vi "OP80FV_Check.vi"(6 "View":bool=TRUE, 8 "error in (no error)":errorcluster, 10 "RFID":string="0029032640C1845Ag000001", 11 "Ref in":T2={"MS SQL Connection"=refnum, "UDL File"=path "", "Time"="", "DCODE"="", "WIP+1"=0, "MC No?"=0, "POKAYOKE?"=FALSE, "Expected Result"="", "Result [Status]"="", "Clock"=0.0, "RFID"="", "WIP Queue"=refnum, "TS Parameter"={"ProfitCenterCode"="", "LineCode"="", "WorkOrderNumber"="", "Model"="", "Model_with_Prefix"="", "VendorCode"="", "SetParameterDateCode"="", "PokaYoke"=0, "Target"=1, "Live_DateCode"="", "CustomerPartNumber"="", "Hand"="", "sBarcode"=FALSE, "FCA"=0, "Ent_Stamp"=timestamp(0 s since 1904-01-01), "STS_CD"=0.0}, "Data_Queue"=[], "RFID Serial No."=""} {"TS Parameter"."FCA" format="%01d"; "TS Parameter"."Target" min=1 max=100000; "TS Parameter"."PokaYoke" min=0 max=1}) -> (0 "error out":errorcluster, 1 "Fail?":bool=TRUE, 2 "Pass?":bool=TRUE, 3 "Ref Out":T2={"MS SQL Connection"=refnum, "UDL File"=path "", "Time"="", "DCODE"="", "WIP+1"=0, "MC No?"=0, "POKAYOKE?"=FALSE, "Expected Result"="", "Result [Status]"="", "Clock"=0.0, "RFID"="", "WIP Queue"=refnum, "TS Parameter"={"ProfitCenterCode"="", "LineCode"="", "WorkOrderNumber"="", "Model"="", "Model_with_Prefix"="", "VendorCode"="", "SetParameterDateCode"="", "PokaYoke"=0, "Target"=1, "Live_DateCode"="", "CustomerPartNumber"="", "Hand"="", "sBarcode"=FALSE, "FCA"=0, "Ent_Stamp"=timestamp(0 s since 1904-01-01), "STS_CD"=0.0}, "Data_Queue"=[], "RFID Serial No."=""} {"TS Parameter"."FCA" format="%01d"; "TS Parameter"."Target" min=1 max=100000; "TS Parameter"."PokaYoke" min=0 max=1}, 4 "Discard?":bool=TRUE, 5 "Reason Out":string, 7 "appended array":string[](array[string]))   [LabVIEW 2020]
uses:
  Controls/TD SQL.ctl
  <vilib>/addons/database/Connection.llb/Conn ObjectReference.ctl
  Controls/WIP_State.ctl
  Controls/TS_Parameter.ctl
  Controls/FV_Status.ctl
  <vilib>/Utility/miscctls.llb/LVPointTypeDef.ctl
  Controls/1775E_Authen_Level.ctl
  Controls/Station_Task.ctl
  MS SQL/MS_Global.vi
  <userlib>/_OpenG.lib/comparison/comparison.llb/Boolean Changed__ogtk.vi
  <userlib>/_OpenG.lib/comparison/comparison.llb/String Changed__ogtk.vi
  <vilib>/addons/database/Connection.llb/Conn Execute.vi
  <vilib>/addons/database/Recordset.llb/Rec Destroy - Connection.vi
  <vilib>/ethernetip/ethernetip.llb/EthernetIP Tag Write DINT.vi
  <vilib>/Utility/miscctls.llb/LVRowAndColumnTypeDef.ctl
  <vilib>/Utility/miscctls.llb/LVRowAndColumnUnsignedTypeDef.ctl
  <vilib>/ethernetip/ethernetip.lvlib
  <vilib>/addons/database/NI_Database_API.lvlib
panel:
  out "resulting string":string
  out "Barcode":string
  out "Text Command for Printer":string
  out "Last Printed BC Mirror":string
  out "Last Printed Barcode":string
  out "Numeric":i32
  in  "Hide":bool
  in  "Reprint":bool
  in  "Scan":bool
  out "OP80 RFID":string
  in  "Fail":bool
  out "Over all Status":T1 caption="Data Validation"
  in  "RH Barcode":string="0029032640C1845Ag000001"
  in  "LH Barcode":string="0029032640C1845Ag000001"
  out "pPASS":bool
  out "pFAIL":bool
  in  "Pass":bool caption="Final Viewing"
  in  "Report":i32(listbox)
  in  "Time to Close":dbl format="%.1f"
  in  "Reason":string
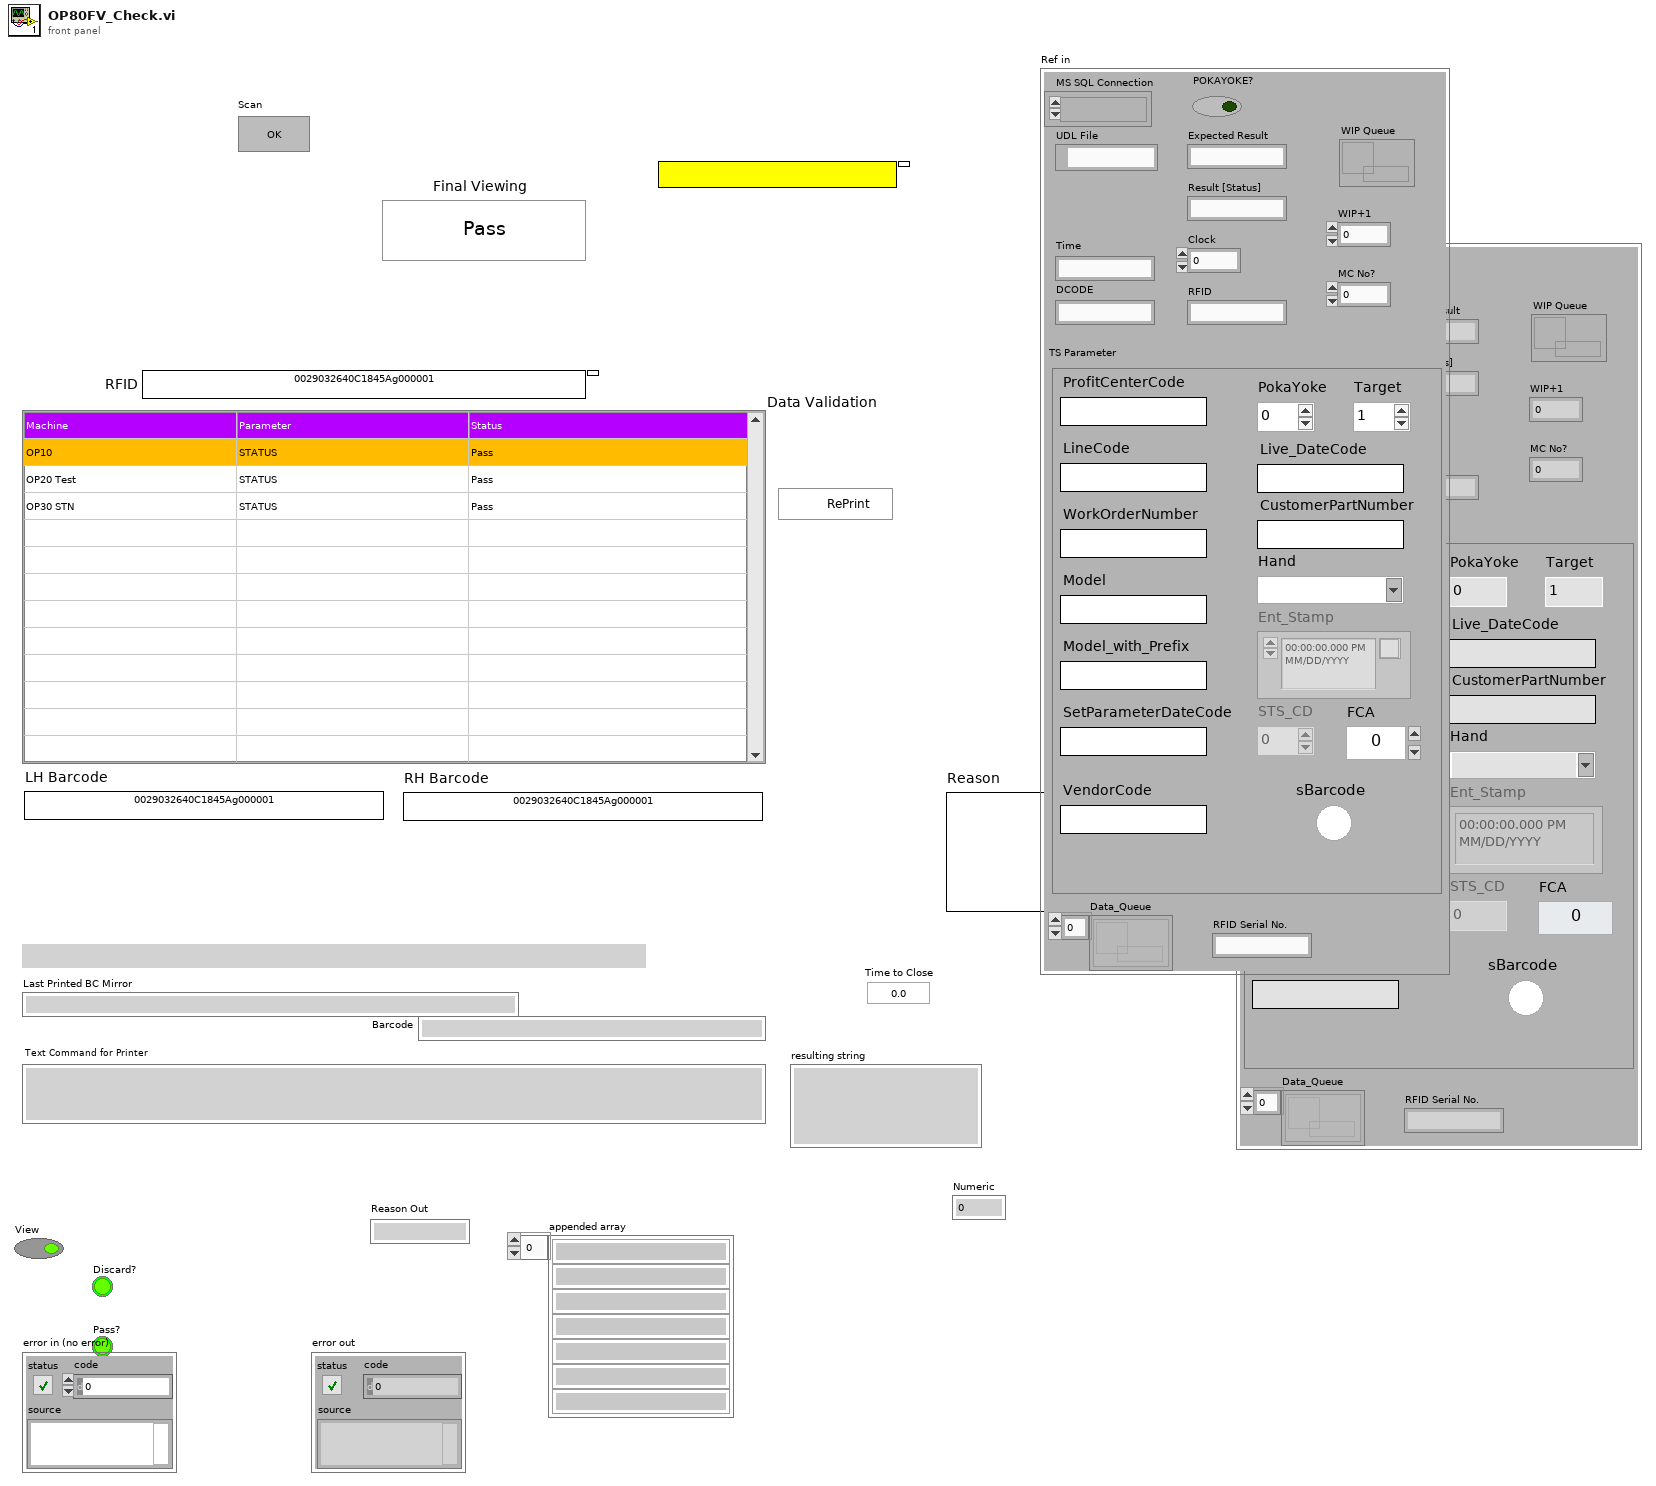
[diagram p1: front panel]
types:
  T1 = typedef "FV_Status.ctl" = u16
  T2 = typedef "TD SQL.ctl" = cluster{"MS SQL Connection":T3, "UDL File":path, "Time":string, "DCODE":string, "WIP+1":i64, "MC No?":i32, "POKAYOKE?":bool, "Expected Result":string, "Result [Status]":string, "Clock":dbl, "RFID":string, "WIP Queue":refnum<queue>, "TS Parameter":T4, "Data_Queue":refnum<queue>[], "RFID Serial No.":string}
  T3 = typedef "NI_Database_API.lvlib/Conn ObjectReference.ctl" = refnum<k1>
  T4 = typedef "TS_Parameter.ctl" = cluster{"ProfitCenterCode":string, "LineCode":string, "WorkOrderNumber":string, "Model":string, "Model_with_Prefix":string, "VendorCode":string, "SetParameterDateCode":string, "PokaYoke":i32, "Target":i32, "Live_DateCode":string, "CustomerPartNumber":string, "Hand":string, "sBarcode":bool, "FCA":i32, "Ent_Stamp":timestamp, "STS_CD":dbl}
  T5 = typedef "LVPointTypeDef.ctl" = cluster{"Horizontal":i16, "Vertical":i16}
  T6 = typedef "1775E_Authen_Level.ctl" = enum16{"Level 1", "Level 2", "Level 3", "Level 4", "Super Level"}
  T7 = typedef "LVRowAndColumnUnsignedTypeDef.ctl" = cluster{"Row":u32, "Column":u32}
  T8 = typedef "LVRowAndColumnTypeDef.ctl" = cluster{"Row":i32, "Column":i32}
  T9 = enum8{"Enabled", "Disabled", "Disabled and Grayed Out"}
  T10 = cluster{"CUSTOMER PART NUMBER":string, "Version Number":string, "VENDOR CODE":string, "BI PART NUMBER":string, "SCAN TYPE":enum16{"AUTO", "MANUAL"}, "BARCODE TYPE":enum16{"X451", "MSIL-YNC10 Trial1"}, "CELL NUMBER":string}
  T11 = typedef "Station_Task.ctl" = enum16{"Init", "Polling", "Check Bypass", "Check_Result", "get Barcode", "Pass", "Fail", "Check Data", "Log Data", "Idle_Alert", "DMS_Check", "FV_Check", "FV_View", "WRITE_RFID", "Exit"}
  T12 = typedef "user_log.ctl" = cluster{"eRID":u16, "eRName":string, "eRClock":string, "eRDate":timestamp, "eRLevel":string, "eRAdmin":string, "eRPassword":string}
  T13 = typedef "NI_Database_API.lvlib/Rec ObjectReference.ctl" = refnum<k1>
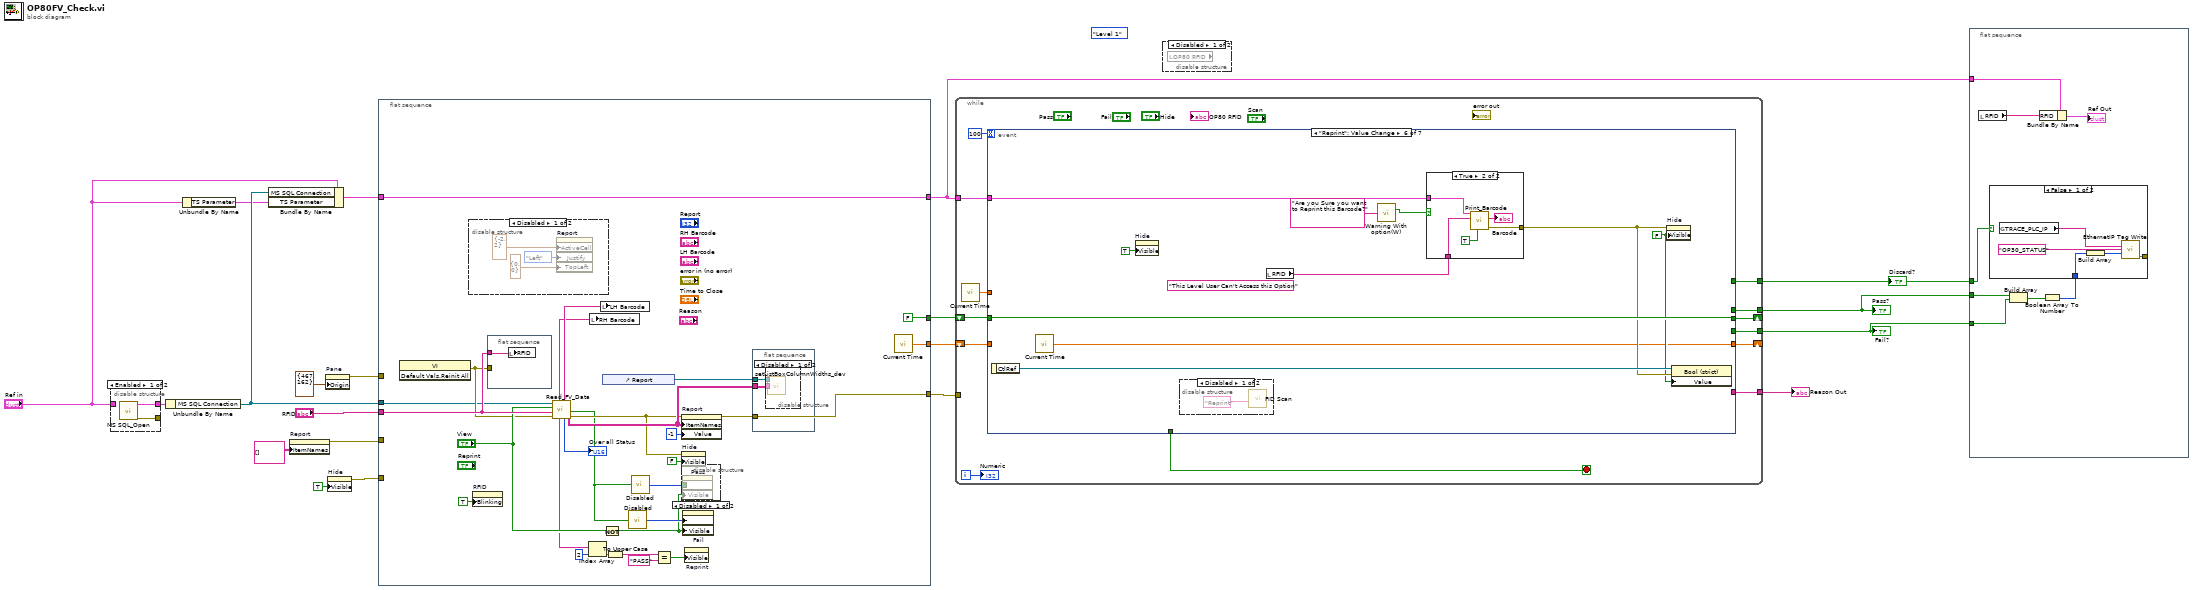
[diagram p0: block diagram]
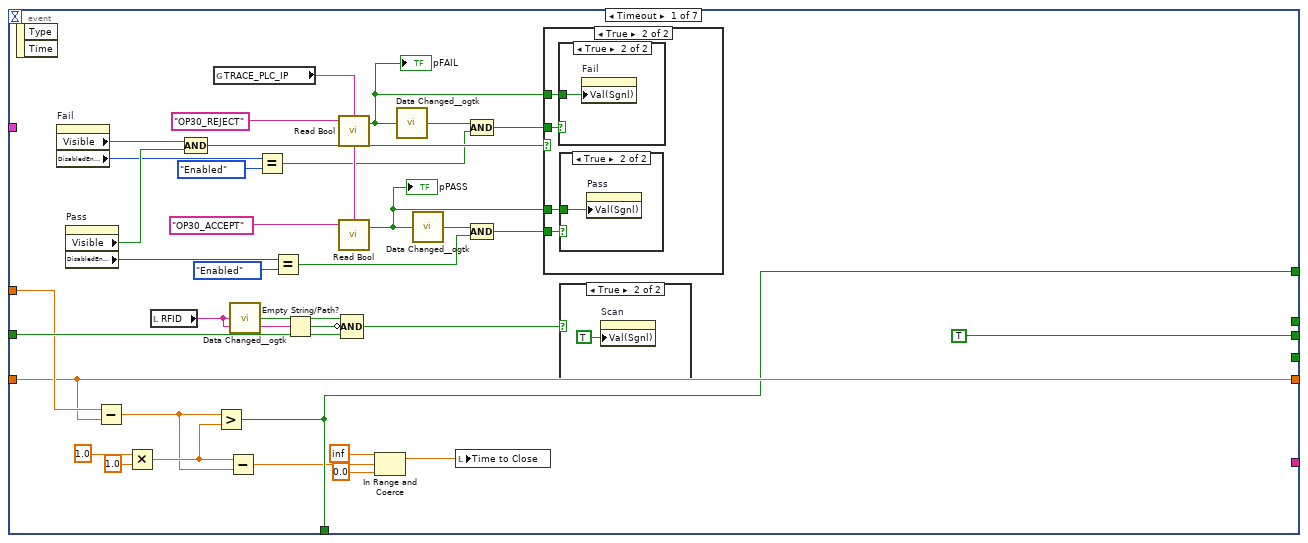
[diagram p8: hidden frame]
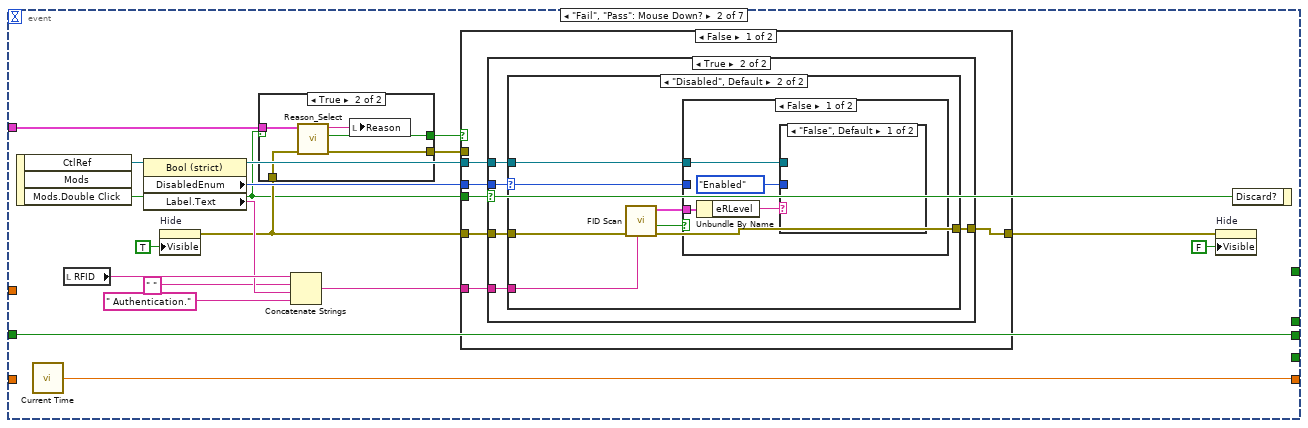
[diagram p13: hidden frame]
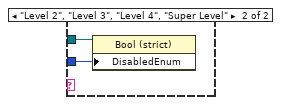
[diagram p17: hidden frame]
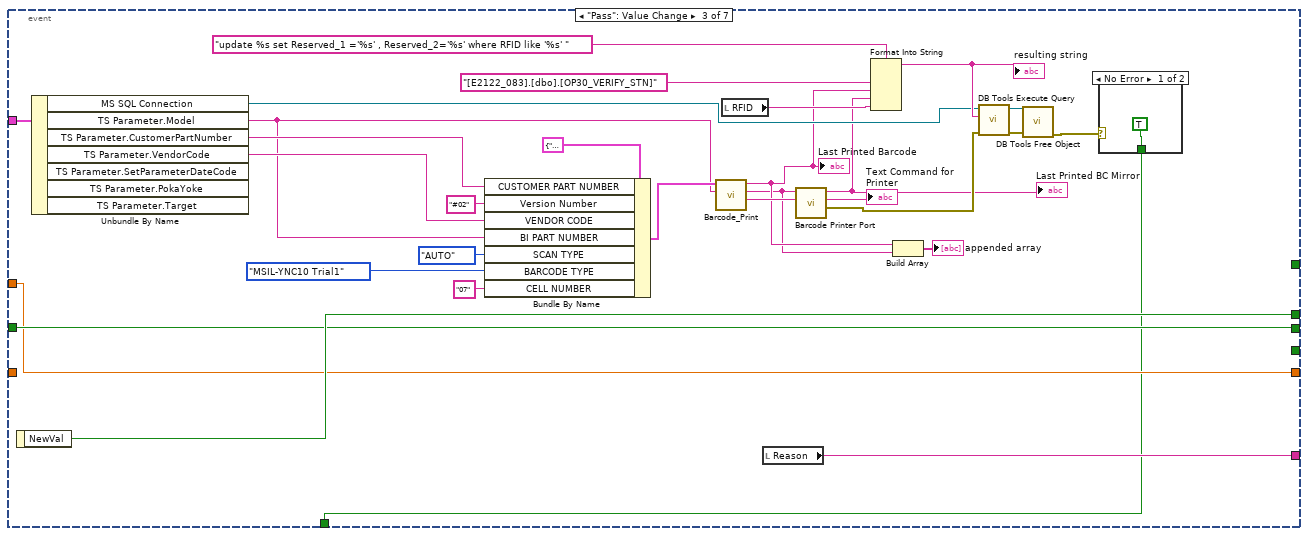
[diagram p20: hidden frame]
diagram:
  (unwired) 1775E_Authen_Level."Level 1" ("Level")
  n1 = disable-structure shown="Enabled" {
    disable-tunnel: [w22 w23] -> w19
    disable-tunnel: "Ref in" -> [_ w23]
    disable-tunnel: [w21 _] -> _
    frame Enabled {
      n2 = call "MS SQL_Open.vi"() -> ("error out"=w21:errorcluster, "Ref Out"=w22:T2)  [unwired: 9 in, 1 out]
    }
    frame Disabled {
    }
  }
  n3 = Unbundle By Name(w19) -> ("MS SQL Connection"=w17:T3)
  n4 = Unbundle By Name("Ref in") -> ("TS Parameter"=w1:T4)
  n5 = Bundle By Name(cluster="Ref in", "MS SQL Connection"=w17, "TS Parameter"=w1) -> (w16:T2)
  n6 = property on="Report" class="MCListbox (strict)"("ItemNames"=string[][] [] ("Item Names")) -> (error out=w6:errorcluster)  [unwired: 2 in, 1 out]
  n7 = property on="Pane" class="Pane"("Origin"=T5 {"Horizontal"=467, "Vertical"=162}) -> (error out=w12:errorcluster)  [unwired: 2 in, 1 out]
  n8 = property on="Hide" class="Bool"("Visible"=TRUE) -> (error out=w3:errorcluster)  [unwired: 2 in, 1 out]
  n9 = flat-sequence {
    tunnel: w17 -> [w40]
    tunnel: [w38] -> w20
    tunnel: w16 -> [w48]
    tunnel: [w48] -> w15
    tunnel: "RFID" -> [w46]
    tunnel: [FALSE ("empty?")] -> w14
    tunnel: w12 -> [_]
    tunnel: [w30] -> w10
    tunnel: w6 -> [_]
    tunnel: w3 -> [_]
    frame #0 {
      n10 = invoke class="VI" method="Default Vals.Reinit All"() -> (error out=w42:errorcluster)  [unwired: 3 in, 2 out]
      n11 = disable-structure shown="Disabled" {
        frame Disabled {
          n12 = property on="Report" class="MCListbox (strict)"("ActiveCell"=T8 {"Row"=-2, "Column"=2} ("Active Cell:Active Cell"), "Justify"=enum16{"Left", "Center", "Right"}."Left" ("Active Cell:Cell Justification"), "TopLeft"=T7 {"Row"=0, "Column"=0} ("Top Left Visible Cell")) -> ()  [unwired: 2 in, 2 out]
        }
        frame Enabled {
        }
      }
      n13 = property on="RFID" class="Str"("Blinking"=TRUE) -> ()  [unwired: 2 in, 2 out]
      n14 = flat-sequence {
        tunnel: w46 -> [w56]
        tunnel: w42 -> [_]
        frame #0 {
          n15 = local write "RFID"(w56) -> ()
        }
      }
      n16 = call "Read_FV_Data.vi"("error in (no error)"=w42, "RFID"=w46, "View"="View", "MS SQL Connection"=w40) -> ("error out"=w26:errorcluster, "Enable?"=w25:bool, "Report"=w39:string[][], "REsult"=→"Over all Status":T1, "Final View Barcode"=w47:string, "All Status"=w35:string[], "ASR Barcode"=w36:string)  [unwired: 1 out]
      n17 = Index Array(array=w35, index=2) -> (element=w33:string)
      n18 = local write "RH Barcode"(w36) -> ()
      n19 = local write "LH Barcode"(w47) -> ()
      n20 = control-ref of="Report"() -> (w50:refnum<vi>)
      n21 = Not(x="View") -> (.not. x?=w29:bool)
      n22 = To Upper Case(1:w33) -> (0:w31:string)
      n23 = call <userlib>:"Disabled.vi"("Enable?"=w25) -> ("Disabled"=w44:T9)  [unwired: 14 in]
      n24 = call <userlib>:"Disabled.vi"("Enable?"=w25) -> ("Disabled"=w45:T9)  [unwired: 14 in]
      n25 = Equal?(x=w31, y="PASS") -> (x = y?=w24:bool)
      n26 = property on="Report" class="MCListbox (strict)"(error in=w26, "ItemNames"=w39, "Value"=-1 ("Multicolumn Listbox")) -> (error out=w38:errorcluster)  [unwired: 1 in, 1 out]
      n27 = property on="Hide" class="Bool"(error in=w26, "Visible"=FALSE) -> ()  [unwired: 1 in, 2 out]
      n28 = disable-structure shown="Disabled" {
        disable-tunnel: w45 -> [w52 _]
        disable-tunnel: w29 -> [w51 _]
        frame Disabled {
          n29 = property on="Pass" class="Bool (strict)"("DisabledEnum"=w52, "Visible"=w51) -> ()  [unwired: 2 in, 2 out]
        }
        frame Enabled {
        }
      }
      n30 = property on="Fail" class="Bool (strict)"("DisabledEnum"=w44, "Visible"=w29) -> ()  [unwired: 2 in, 2 out]
      n31 = property on="Reprint" class="Bool (strict)"("Visible"=w24) -> ()  [unwired: 2 in, 2 out]
      n32 = flat-sequence {
        tunnel: w39 -> [w58]
        tunnel: w50 -> [w57]
        tunnel: w38 -> [_]
        frame #0 {
          n33 = disable-structure shown="Disabled" {
            disable-tunnel: w58 -> [w60 _]
            disable-tunnel: w57 -> [w59 _]
            frame Disabled {
              n34 = call "setListBoxColumnWidths_dev.vi"("table data"=w60, "MCListbox Refnum"=w59) -> ()  [unwired: 1 in]
            }
            frame Enabled {
            }
          }
        }
      }
      n35 = call <userlib>:"Current Time.vi"() -> ("Current Time (Sec)"=w30:dbl)  [unwired: 15 in]
    }
  }
  n36 = while {
    tunnel: w20 -> [_]
    tunnel: [w72] -> w11
    tunnel: [w71] -> w9
    tunnel: [w70] -> w8
    tunnel: w15 -> [w66]
    shift-right: [w67] -> _
    shift-left: w14 -> [w68]
    shift-right: [w64] -> _
    shift-left: w10 -> [w65]
    tunnel: [w62] -> w7
    i -> [w61]
    stop <- w73 stop-if-true
    n37 = call <userlib>:"Current Time.vi"() -> ("Current Time (Sec)"=w63:dbl)  [unwired: 15 in]
    n38 = event shown="[5] \"Reprint\": Value Change" {
      selector: _ -> [_ _ _ _ _ _ _]
      dyn-events: _ -> [_ _ _ _ _ _ _]
      timeout: 100 -> [_ _ _ _ _ _ _]
      tunnel: [w91 _ w167 w197 _ _ w263] -> w73
      tunnel: [w91 _ _ _ _ _ w263] -> w72
      tunnel: [_ _ w191 _ _ _ _] -> w71
      tunnel: [_ _ _ w197 _ _ _] -> w70
      tunnel: w68 -> [w98 w128 w190 w196 w231 w253 w262]
      tunnel: [TRUE ("empty?") w128 w190 w196 w231 w253 w262] -> w67
      tunnel: w66 -> [_ w121 w186 _ w230 w251 _]
      tunnel: w65 -> [w94 _ _ _ _ _ w261]
      tunnel: [w94 w125 w189 w195 w206 w245 w261] -> w64
      tunnel: w63 -> [w95 _ w189 w195 w206 _ _]
      tunnel: [_ _ w188 w194 _ _ _] -> w62
      event Timeout {
        n39 = event-data() -> ()  [unwired: 1 in, 2 out]
        n40 = property on="Fail" class="Bool (strict)"() -> ("Visible"=w83:bool, "DisabledEnum"=w81:T9)  [unwired: 2 in, 2 out]
        n41 = property on="Pass" class="Bool (strict)"() -> ("Visible"=w84:bool, "DisabledEnum"=w75:T9)  [unwired: 2 in, 2 out]
        n42 = Subtract(x=w95, y=w94) -> (x-y=w89:dbl)
        n43 = Multiply(x=1.0, y=1.0) -> (x*y=w90:dbl)
        n44 = local read "RFID"() -> (w100:string)
        n45 = Compound Arithmetic op=AND(w83, w84) -> (w82:bool)
        n46 = global read "MS_Global.vi" "TRACE_PLC_IP"() -> (w106:string)
        n47 = Greater?(x=w89, y=w90) -> (0:w91:bool)
        n48 = Subtract(x=w90, y=w89) -> (x-y=w86:dbl)
        n49 = call-poly <userlib>:"Data Changed__ogtk.vi"("String"=w100) -> ("Changed"=w101:bool)
        n50 = Equal?(x=w81, y=T9."Enabled") -> (x = y?=w78:bool)
        n51 = Equal?(x=w75, y=T9."Enabled") -> (x = y?=w74:bool)
        n52 = Empty String/Path?(string/path=w100) -> (empty?=w99:bool)
        n53 = call "Read Bool.vi"("Network Path"=w106, "Tag Name"="OP30_REJECT") -> ("BOOL"=w103:bool)  [unwired: 3 in]
        "pFAIL" <- w103
        n54 = call "Read Bool.vi"("Network Path"=w106, "Tag Name"="OP30_ACCEPT") -> ("BOOL"=w102:bool)  [unwired: 3 in]
        "pPASS" <- w102
        n55 = Compound Arithmetic op=AND(w101, invert w99, w98) -> (w96:bool)
        n56 = In Range and Coerce(upper limit=inf, x=w86, lower limit=0.0) -> (coerced(x)=w85:dbl)  [unwired: 1 out]
        n57 = call-poly <userlib>:"Data Changed__ogtk.vi"("Boolean"=w103) -> ("Changed"=w105:bool)
        n58 = call-poly <userlib>:"Data Changed__ogtk.vi"("Boolean"=w102) -> ("Changed"=w104:bool)
        n59 = local write "Time to Close"(w85) -> ()
        n60 = Compound Arithmetic op=AND(w105, w78) -> (w79:bool)
        n61 = Compound Arithmetic op=AND(w104, w74) -> (w77:bool)
        n62 = case shown="True" w82 {
          tunnel: w79 -> [_ w112]
          tunnel: w77 -> [_ w111]
          tunnel: w103 -> [_ w110]
          tunnel: w102 -> [_ w109]
          frame False {
          }
          frame True {
            n63 = case shown="True" w112 {
              tunnel: w110 -> [_ w114]
              frame False {
              }
              frame True {
                n64 = property on="Fail" class="Bool (strict)"("Val(Sgnl)"=w114) -> ()  [unwired: 2 in, 2 out]
              }
            }
            n65 = case shown="True" w111 {
              tunnel: w109 -> [_ w113]
              frame False {
              }
              frame True {
                n66 = property on="Pass" class="Bool (strict)"("Val(Sgnl)"=w113) -> ()  [unwired: 2 in, 2 out]
              }
            }
          }
        }
        n67 = case shown="True" w96 {
          frame False {
          }
          frame True {
            n68 = property on="Scan" class="Bool (strict)"("Val(Sgnl)"=TRUE ("Value (Signaling)")) -> ()  [unwired: 2 in, 2 out]
          }
        }
      }
      event "Fail", "Pass": Mouse Down? {
        n69 = event-data() -> ("CtlRef"=w130:refnum<vi>, "Mods.Double Click"=w116:bool)  [unwired: 1 in, 1 out]
        n70 = call <userlib>:"Current Time.vi"() -> ("Current Time (Sec)"=w125:dbl)  [unwired: 15 in]
        n71 = local read "RFID"() -> (w124:string)
        n72 = property class="Bool (strict)"(reference=w130) -> (reference out=w133:refnum<vi>, "DisabledEnum"=w132:T9, "Label.Text"=w123:string)  [unwired: 1 in, 1 out]
        n73 = property on="Hide" class="Bool"("Visible"=TRUE) -> (error out=w119:errorcluster)  [unwired: 2 in, 1 out]
        n74 = case shown="True" w116 {
          tunnel: w121 -> [_ w138]
          tunnel: w119 -> [_ w136]
          tunnel: [_ w135] -> w118
          tunnel: [_ w134] -> w117
          frame False {
          }
          frame True {
            n75 = call "Reason_Select.vi"("error in (no error)"=w136, "Ref in"=w138) -> ("error out"=w134:errorcluster, "Cancel?"=w135:bool, "Reason Out"=w137:string)  [unwired: 7 in]
            n76 = local write "Reason"(w137) -> ()
          }
        }
        n77 = Concatenate Strings(w124, " " ("string"), w123, " Authentication." ("string")) -> (w126:string)
        n78 = case shown="False" w118 {
          tunnel: w133 -> [w144 _]
          tunnel: w132 -> [w143 _]
          tunnel: [w142 w163] -> w129
          tunnel: w116 -> [w141 _]
          tunnel: w126 -> [w140 _]
          tunnel: w119 -> [w139 w163]
          tunnel: w117 -> [_ _]
          frame False {
            n79 = case shown="True" w141 {
              tunnel: [_ w149] -> w142
              tunnel: w144 -> [_ w148]
              tunnel: w143 -> [_ w147]
              tunnel: w140 -> [_ w146]
              tunnel: w139 -> [_ w145]
              frame False {
              }
              frame True {
                n80 = case shown="\"Disabled\", Default" w147 {
                  selector: w147 -> [_ w152]
                  tunnel: [_ w156] -> w149
                  tunnel: w148 -> [_ w154]
                  tunnel: w146 -> [_ w151]
                  tunnel: w145 -> [_ w150]
                  frame "Enabled" {
                  }
                  frame "Disabled", Default {
                    n81 = call "FID Scan.vi"("Purpose"=w151, "error in (no error)"=w150) -> ("error out"=w156:errorcluster, "Cancel ?"=w155:bool, "data"=w153:T12)  [unwired: 7 in]
                    n82 = case shown="False" w155 {
                      tunnel: w154 -> [w158 _]
                      tunnel: w153 -> [w160 _]
                      tunnel: w152 -> [_ _]
                      frame False {
                        n83 = Unbundle By Name(w160) -> ("eRLevel"=w159:string)
                        n84 = case shown="\"False\", Default" w159 {
                          tunnel: w158 -> [_ w162]
                          tunnel: T9."Enabled" ("Disabled") -> [_ w161]
                          frame "False", Default {
                          }
                          frame "Level 2", "Level 3", "Level 4", "Super Level" {
                            n85 = property class="Bool (strict)"(reference=w162, "DisabledEnum"=w161) -> ()  [unwired: 1 in, 2 out]
                          }
                        }
                      }
                      frame True {
                      }
                    }
                  }
                }
              }
            }
          }
          frame True {
          }
        }
        n86 = property on="Hide" class="Bool"(error in=w129, "Visible"=FALSE) -> ()  [unwired: 1 in, 2 out]
        n87 = event-data("Discard?"=w116) -> ()  [unwired: 1 in, 1 out]
      }
      event "Pass": Value Change {
        n88 = event-data() -> ("NewVal"=w191:bool)  [unwired: 1 in]
        n89 = Unbundle By Name(w186) -> ("MS SQL Connection"=w172:T3, "TS Parameter.Model"=w181:string, "TS Parameter.CustomerPartNumber"=w183:string, "TS Parameter.VendorCode"=w182:string)  [unwired: 3 out]
        n90 = Bundle By Name(cluster=T10 {"CUSTOMER PART NUMBER"="106", "Version Number"="106", "VENDOR CODE"="106", "BI PART NUMBER"="106", "SCAN TYPE"=enum."AUTO", "BARCODE TYPE"=enum."X451", "CELL NUMBER"=""} ("Parameter"), "CUSTOMER PART NUMBER"=w183, "Version Number"="#02", "VENDOR CODE"=w182, "BI PART NUMBER"=w181, "SCAN TYPE"=enum16{"AUTO", "MANUAL"}."AUTO", "BARCODE TYPE"=enum16{"X451", "MSIL-YNC10 Trial1"}."MSIL-YNC10 Trial1", "CELL NUMBER"="07") -> (w184:T10)
        n91 = call "Barcode_Print"("Ring Text.Text"=w181, "Parameter"=w184) -> ("Text Command for Printer"=w187:string, "Last Printed BC Mirror"=w165:string, "Last Printed Barcode"=w166:string)  [unwired: 7 in]
        "Last Printed Barcode" <- w166
        "Last Printed BC Mirror" <- w165
        "Text Command for Printer" <- w187
        n92 = local read "RFID"() -> (w174:string)
        n93 = local read "Reason"() -> (w188:string)
        n94 = call "Barcode Printer Port.vi"("string to write"=w187) -> ("error out"=w171:errorcluster)  [unwired: 10 in]
        n95 = Format Into String(format string="update %s set Reserved_1 ='%s' , Reserved_2='%s' where RFID like '%s' " ("condition"), "[E2122_083].[dbo].[OP30_VERIFY_STN]" ("table"), w166, w165, w174) -> (resulting string=w173:string)  [unwired: 2 in, 1 out]
        "resulting string" <- w173
        n96 = Build Array(w166, w165) -> (→"appended array":string[])
        n97 = call-poly <vilib>:"DB Tools Execute Query.vi"("error in (no error)"=w171, "SQL query"=w173, "connection reference"=w172) -> ("error out"=w170:errorcluster, "recordset reference"=w169:T13)  [unwired: 5 in]
        n98 = call-poly <vilib>:"DB Tools Free Object.vi"("error in (no error)"=w170, "recordset reference"=w169) -> ("error out"=w168:errorcluster)  [unwired: 8 in, 1 out]
        n99 = case shown="No Error" w168 {
          tunnel: [TRUE ("Discard?") FALSE ("Discard?")] -> w167
          frame No Error {
          }
          frame Error {
          }
        }
      }
      event "Fail": Value Change {
        n100 = event-data() -> ("NewVal"=w197:bool)  [unwired: 1 in]
        n101 = local read "Reason"() -> (w194:string)
      }
      event "Scan": Value Change {
        n102 = event-data() -> ("CtlRef"=w201:refnum<vi>)  [unwired: 1 in]
        n103 = local read "RFID"() -> (w226:string)
        n104 = property on="Hide" class="Bool"("Visible"=TRUE) -> (error out=w203:errorcluster)  [unwired: 2 in, 1 out]
        n105 = Bundle By Name(cluster=w230, "RFID"=w226, "MC No?"=2) -> (w229:T2)
        n106 = local write "RFID"(w226) -> ()
        n107 = call "RFID_Checker.vi"("error in (no error)"=w203, "Ref in"=w229) -> ("error out"=w224:errorcluster, "TS_BSC"=w227:i32, "Ref out"=w225:T2)  [unwired: 5 in, 2 out]
        n108 = Unbundle By Name(w225) -> ("MS SQL Connection"=w223:T3)
        n109 = case shown="0, Default" w227 {
          tunnel: [Station_Task."FV_Check" ("Enum") w239] -> _
          tunnel: w226 -> [_ w243]
          tunnel: [FALSE ("empty?") TRUE ("empty?")] -> w215
          tunnel: w224 -> [w235 _]
          tunnel: [w234 _] -> w222
          frame 1 {
            n110 = call <vilib>:"Clear Errors.vi"("error in (no error)"=w235) -> ("error out"=w234:errorcluster)  [unwired: 5 in, 1 out]
          }
          frame 0, Default {
            n111 = Empty String/Path?(string/path=w243) -> (empty?=w242:bool)
            n112 = Select(t=Station_Task."Polling" ("Enum"), s=w242, f=Station_Task."FV_View") -> (s? t:f=w239:T11)
          }
        }
        n113 = call "Read_FV_Data.vi"("error in (no error)"=w222, "RFID"=w226, "View"=w215, "MS SQL Connection"=w223) -> ("error out"=w200:errorcluster, "Enable?"=w216:bool, "Report"=w213:string[][], "REsult"=w220:T1, "Final View Barcode"=w221:string, "All Status"=w207:string[], "ASR Barcode"=w212:string)  [unwired: 1 out]
        n114 = local write "RH Barcode"(w212) -> ()
        n115 = local write "Over all Status"(w220) -> ()
        n116 = local write "LH Barcode"(w221) -> ()
        n117 = Not(x=w216) -> (.not. x?=w205:bool)
        n118 = Not(x=w215) -> (.not. x?=w217:bool)
        n119 = Index Array(array=w207, index=11) -> (element=w209:string)
        n120 = call <userlib>:"Disabled.vi"("Enable?"=w205) -> ("Disabled"=w218:T9)  [unwired: 14 in]
        n121 = call <userlib>:"Disabled.vi"("Enable?"=w216) -> ("Disabled"=w219:T9)  [unwired: 14 in]
        n122 = To Upper Case(1:w209) -> (0:w211:string)
        n123 = property on="Hide" class="Bool"(error in=w200, "Visible"=FALSE) -> ()  [unwired: 1 in, 2 out]
        n124 = disable-structure shown="Disabled" {
          disable-tunnel: w219 -> [w233 _]
          disable-tunnel: w217 -> [w232 _]
          frame Disabled {
            n125 = property on="Pass" class="Bool (strict)"("DisabledEnum"=w233, "Visible"=w232) -> ()  [unwired: 2 in, 2 out]
          }
          frame Enabled {
          }
        }
        n126 = Equal?(x=w211, y="PASS") -> ()  [unwired: 1 out]
        n127 = property on="Fail" class="Bool (strict)"("DisabledEnum"=w218, "Visible"=w217) -> ()  [unwired: 2 in, 2 out]
        n128 = property on="Reprint" class="Bool (strict)"("Visible"=TRUE) -> ()  [unwired: 2 in, 2 out]
        n129 = property class="Bool (strict)"(reference=w201, error in=w200, "Value"=FALSE) -> ()  [unwired: 2 out]
        n130 = property on="Report" class="MCListbox (strict)"("ItemNames"=w213, "Value"=-1 ("Multicolumn Listbox")) -> ()  [unwired: 2 in, 2 out]
      }
      event "Reprint": Value Change {
        w246 = FALSE ("Visible")
        (unwired) "This Level User Can't Access this Option" ("Warning in")
        n131 = event-data() -> ("CtlRef"=w248:refnum<vi>)  [unwired: 1 in]
        n132 = call <userlib>:"Current Time.vi"() -> ("Current Time (Sec)"=w245:dbl)  [unwired: 15 in]
        n133 = property on="Hide" class="Bool"("Visible"=TRUE) -> ()  [unwired: 2 in, 2 out]
        n134 = disable-structure shown="Disabled" {
          frame Disabled {
            n135 = call "FID Scan.vi"("Purpose"="Reprint") -> ()  [unwired: 8 in, 3 out]
          }
          frame Enabled {
          }
        }
        n136 = local read "RFID"() -> (w250:string)
        n137 = call <userlib>:"Warning With option(W).vi"("Warning in"="Are you Sure you want to Reprint this Barcode?") -> ("OK 2"=w244:bool)  [unwired: 13 in, 1 out]
        n138 = case shown="True" w244 {
          tunnel: w251 -> [_ w259]
          tunnel: w250 -> [_ w258]
          tunnel: [errorcluster {"status"=FALSE, "code"=0, "source"=""} ("error out") w257] -> w247
          frame False {
          }
          frame True {
            n139 = call "Print_Barcode.vi"("RePrint"=TRUE, "RFID"=w258, "Ref in"=w259) -> ("error out"=w257:errorcluster, "Barcode"=→"Barcode":string)  [unwired: 2 in, 5 out]
          }
        }
        n140 = property on="Hide" class="Bool"(error in=w247, "Visible"=w246) -> ()  [unwired: 1 in, 2 out]
        n141 = property class="Bool (strict)"(reference=w248, error in=w247, "Value"=w246) -> ()  [unwired: 2 out]
      }
      event Panel Close? {
        w263 = TRUE ("Discard?")
        n142 = event-data() -> ()  [unwired: 1 in, 3 out]
        n143 = event-data("Discard?"=w263) -> ()  [unwired: 1 in, 1 out]
      }
    }
    "Numeric" <- w61
  }
  "Discard?" <- w11
  "Pass?" <- w9
  "Fail?" <- w8
  "Reason Out" <- w7
  n144 = disable-structure shown="Disabled" {
    frame Disabled {
      n145 = local read "OP80 RFID"() -> ()  [unwired: 1 out]
    }
    frame Enabled {
    }
  }
  n146 = flat-sequence {
    tunnel: w15 -> [w271]
    tunnel: w11 -> [w264]
    tunnel: w9 -> [w267]
    tunnel: w8 -> [w266]
    frame #0 {
      n147 = local read "RFID"() -> (w269:string)
      n148 = Build Array(w267, w266) -> (w268:bool[])
      n149 = Bundle By Name(cluster=w271, "RFID"=w269) -> (→"Ref Out":T2)
      n150 = Boolean Array To Number(Boolean array=w268) -> (number=w265:u32)
      n151 = case shown="False" w264 {
        tunnel: w265 -> [w273 _]
        tunnel: [w272 _] -> _
        frame False {
          n152 = global read "MS_Global.vi" "TRACE_PLC_IP"() -> (w276:string)
          n153 = Build Array(w273) -> (w274:u32[])
          n154 = call-poly <vilib>:"EthernetIP Tag Write.vi"("Network Path"=w276, "Tag Name"="OP30_STATUS" ("Network Path"), "Data"=w274) -> ("error out"=w272:errorcluster)  [unwired: 11 in, 1 out]
        }
        frame True {
        }
      }
    }
  }
